vi "Load Config Data MHL CODE.vi"(8 "error in (no error)":errorcluster, 11 "Settings in":refnum<class "Settings.lvclass">) -> (0 "error out":errorcluster, 2 "Config Data":T1={"DS First Launch"=FALSE, "LogBaseFolder"=path "", "Live Logging"=FALSE, "Server Port"=0, "Max Number ML Rows"=0, "AM.WinBounds"={"Left"=0, "Top"=0, "Right"=0, "Bottom"=0}, "AM.FP.State"=enum."Invalid", "AM.Monitor"=0, "AM.Column Widths"=[], "ML.Visible Columns"=[], "ML.Splitter Position"=0, "ML.Column Widths"=[], "ML.WinBounds"={"Left"=0, "Top"=0, "Right"=0, "Bottom"=0}, "ML.FP.State"=enum."Invalid", "ML.Monitor"=0}, 3 "Settings out":refnum<class "Settings.lvclass">)   [LabVIEW 2017, in "Settings.lvclass"]
uses:
  Settings.lvclass
  Config Data.ctl
  <vilib>/Utility/miscctls.llb/LVRectTypeDef.ctl
  <vilib>/Utility/miscctls.llb/LVAllMonitorsDisplayTypeDef.ctl
  <vilib>/Utility/config.llb/Read Key (Boolean).vi
  <vilib>/Utility/config.llb/Read Key (Path).vi
  <vilib>/Utility/config.llb/Read Key (U32).vi
  <vilib>/Utility/config.llb/Read Key (String).vi
  <vilib>/Utility/config.llb/Read Key (I32).vi
  <vilib>/Utility/config.llb/NI_LVConfig.lvlib
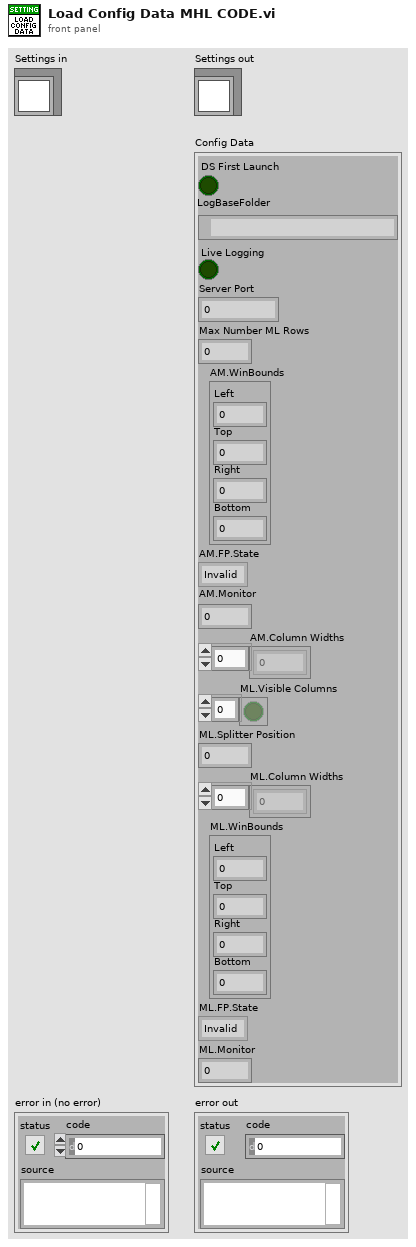
[diagram p1: front panel]
types:
  T1 = typedef "Settings.lvclass/Config Data.ctl" = cluster{"DS First Launch":bool, "LogBaseFolder":path, "Live Logging":bool, "Server Port":u16, "Max Number ML Rows":i32, "AM.WinBounds":T2, "AM.FP.State":enum32{"Invalid", "Standard", "Closed", "Hidden", "Minimized", "Maximized"}, "AM.Monitor":u16, "AM.Column Widths":u32[], "ML.Visible Columns":bool[], "ML.Splitter Position":i32, "ML.Column Widths":u32[], "ML.WinBounds":T2, "ML.FP.State":enum32{"Invalid", "Standard", "Closed", "Hidden", "Minimized", "Maximized"}, "ML.Monitor":u16}
  T2 = typedef "LVRectTypeDef.ctl" = cluster{"Left":i16, "Top":i16, "Right":i16, "Bottom":i16}
  T3 = enum32{"Invalid", "Standard", "Closed", "Hidden", "Minimized", "Maximized"}
  T4 = typedef "LVAllMonitorsDisplayTypeDef.ctl" = cluster{"Bounds":cluster{"Left":i16, "Top":i16, "Right":i16, "Bottom":i16}, "Depth":i16}[]
  T5 = typedef "NI_LVConfig.lvlib/Config Data RefNum.ctl" = refnum<k1>
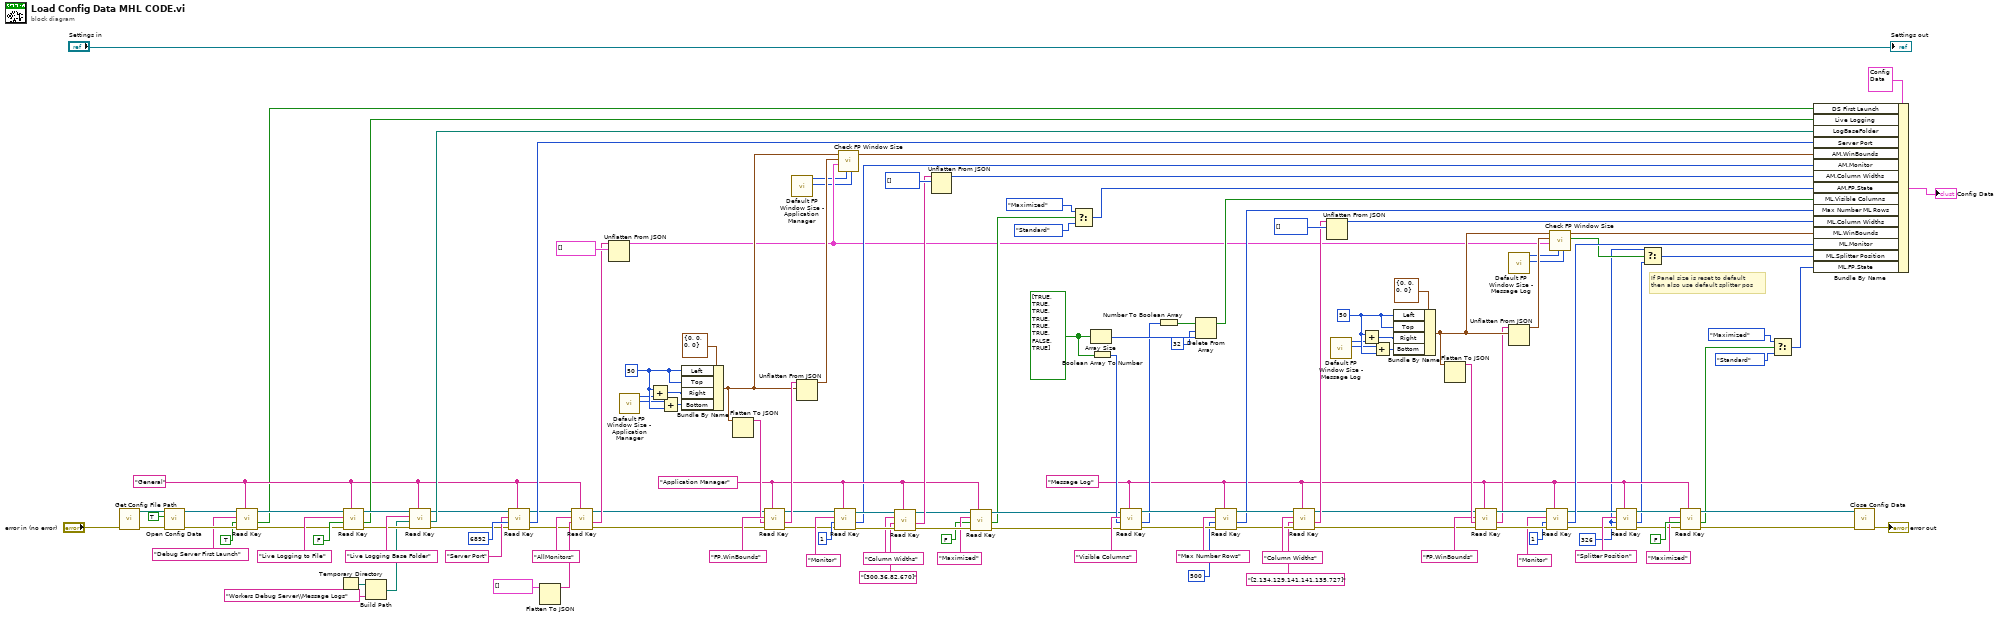
[diagram p0: block diagram]
diagram:
  w11 = 326 ("Splitter Position")
  w39 = i16 50 ("Height")
  w91 = bool[] [TRUE, TRUE, TRUE, TRUE, TRUE, TRUE, FALSE, TRUE] ("Removed ML Columns")
  w105 = i16 50 ("Height")
  w13 = "Message Log" ("section")
  w67 = "Application Manager" ("section")
  w4 = "General" ("section")
  # "If Panel size is reset to default\nthen also use default splitter pos"
  n1 = call "Get Config File Path.vi"("error in (no error)"="error in (no error)") -> ("error out"=w128:errorcluster, "appended path"=w129:path)  [unwired: 9 in]
  n2 = call <vilib>:"Open Config Data.vi"("error in (no error)"=w128, "create file if necessary (T)"=TRUE, "configuration file path"=w129) -> ("error out"=w7:errorcluster, "refnum"=w8:T5)  [unwired: 6 in, 1 out]
  n3 = call-poly <vilib>:"Read Key.vi"("section"=w4, "error in (no error)"=w7, "default value"=TRUE, "key"="Debug Server First Launch" ("name or relative path"), "refnum"=w8) -> ("error out"=w5:errorcluster, "value"=w1:bool, "refnum out"=w6:T5)  [unwired: 3 in, 1 out]
  n4 = Temporary Directory() -> (w119:path)
  n5 = call-poly <vilib>:"Read Key.vi"("section"=w4, "error in (no error)"=w5, "default value"=FALSE, "key"="Live Logging to File", "refnum"=w6) -> ("error out"=w125:errorcluster, "value"=w112:bool, "refnum out"=w126:T5)  [unwired: 3 in, 1 out]
  n6 = Build Path(base path=w119, name or relative path="Workers Debug Server\\Message Logs") -> (appended path=w118:path)
  n7 = call-poly <vilib>:"Read Key.vi"("section"=w4, "error in (no error)"=w125, "default value"=w118, "key"="Live Logging Base Folder", "refnum"=w126) -> ("error out"=w107:errorcluster, "value"=w111:path, "refnum out"=w108:T5)  [unwired: 3 in, 1 out]
  n8 = call-poly <vilib>:"Read Key.vi"("section"=w4, "error in (no error)"=w107, "default value"=u32 6892, "key"="Server Port", "refnum"=w108) -> ("error out"=w55:errorcluster, "value"=w106:u32, "refnum out"=w56:T5)  [unwired: 3 in, 1 out]
  n9 = Flatten To JSON(anything=T4 [] ("Display:All Monitors")) -> (JSON string=w115:string)  [unwired: 2 in, 1 out]
  n10 = call-poly <vilib>:"Read Key.vi"("section"=w4, "error in (no error)"=w55, "default value"=w115, "key"="AllMonitors", "refnum"=w56) -> ("error out"=w54:errorcluster, "value"=w96:string, "refnum out"=w53:T5)  [unwired: 3 in, 1 out]
  n11 = Unflatten From JSON(JSON string=w96, type and defaults=T4 [] ("Display:All Monitors")) -> (value=w25:T4)  [unwired: 5 in, 1 out]
  n12 = call "Default FP Window Size - Application Manager.vi"() -> ("Height"=w101:i16, "Width"=w103:i16)  [unwired: 10 in]
  n13 = Add(x=w105, y=w103) -> (x+y=w104:i16)
  n14 = Add(x=w101, y=w105) -> (x+y=w102:i16)
  n15 = Bundle By Name(cluster=T2 {"Left"=0, "Top"=0, "Right"=0, "Bottom"=0} ("output cluster"), "Left"=w105, "Top"=w105, "Right"=w104, "Bottom"=w102) -> (w68:T2)
  n16 = Flatten To JSON(anything=w68) -> (JSON string=w99:string)  [unwired: 2 in, 1 out]
  n17 = call-poly <vilib>:"Read Key.vi"("section"=w67, "error in (no error)"=w54, "default value"=w99, "key"="FP.WinBounds", "refnum"=w53) -> ("error out"=w52:errorcluster, "value"=w97:string, "refnum out"=w51:T5)  [unwired: 3 in, 1 out]
  n18 = call "Default FP Window Size - Application Manager.vi"() -> ("Height"=w23:i16, "Width"=w24:i16)  [unwired: 10 in]
  n19 = Unflatten From JSON(JSON string=w97, type and defaults=w68) -> (value=w69:T2)  [unwired: 5 in, 1 out]
  n20 = call-poly <vilib>:"Read Key.vi"("section"=w67, "error in (no error)"=w52, "default value"=1 ("Splitter Position"), "key"="Monitor", "refnum"=w51) -> ("error out"=w88:errorcluster, "value"=w65:i32, "refnum out"=w87:T5)  [unwired: 3 in, 1 out]
  n21 = call "Check FP Window Size.vi"("Default Height"=w23, "Default Width"=w24, "All Monitors Display"=w25, "FP.WinBounds"=w69, "Default"=w68) -> ("FP.WinBounds out"=w66:T2)  [unwired: 5 in, 1 out]
  n22 = call-poly <vilib>:"Read Key.vi"("section"=w67, "error in (no error)"=w88, "default value"="[300,36,82,670]", "key"="Column Widths", "refnum"=w87) -> ("error out"=w78:errorcluster, "value"=w81:string, "refnum out"=w76:T5)  [unwired: 3 in, 1 out]
  n23 = Unflatten From JSON(JSON string=w81, type and defaults=u32[] [] ("Column Widths")) -> (value=w64:u32[])  [unwired: 5 in, 1 out]
  n24 = call-poly <vilib>:"Read Key.vi"("section"=w67, "error in (no error)"=w78, "default value"=FALSE, "key"="Maximized", "refnum"=w76) -> ("error out"=w77:errorcluster, "value"=w72:bool, "refnum out"=w75:T5)  [unwired: 3 in, 1 out]
  n25 = Select(t=T3."Maximized" ("y"), s=w72, f=T3."Standard" ("y")) -> (s? t:f=w63:T3)
  n26 = Array Size(array=w91) -> (size(s)=w94:i32)
  n27 = Boolean Array To Number(Boolean array=w91) -> (number=w90:u32)
  n28 = call-poly <vilib>:"Read Key.vi"("section"=w13, "error in (no error)"=w77, "default value"=w90, "key"="Visible Columns", "refnum"=w75) -> ("error out"=w123:errorcluster, "value"=w89:u32, "refnum out"=w124:T5)  [unwired: 3 in, 1 out]
  n29 = Number To Boolean Array(number=w89) -> (Boolean array=w93:bool[])
  n30 = Delete From Array(array=w93, length=32, index=w94) -> (array with subset deleted=w62:bool[])  [unwired: 1 out]
  n31 = call-poly <vilib>:"Read Key.vi"("section"=w13, "error in (no error)"=w123, "default value"=500, "key"="Max Number Rows", "refnum"=w124) -> ("error out"=w83:errorcluster, "value"=w61:i32, "refnum out"=w84:T5)  [unwired: 3 in, 1 out]
  n32 = call-poly <vilib>:"Read Key.vi"("section"=w13, "error in (no error)"=w83, "default value"="[2,134,129,141,141,135,727]", "key"="Column Widths", "refnum"=w84) -> ("error out"=w34:errorcluster, "value"=w79:string, "refnum out"=w33:T5)  [unwired: 3 in, 1 out]
  n33 = Unflatten From JSON(JSON string=w79, type and defaults=u32[] [] ("Column Widths")) -> (value=w60:u32[])  [unwired: 5 in, 1 out]
  n34 = call "Default FP Window Size - Message Log.vi"() -> ("Height"=w21:i16, "Width"=w22:i16)  [unwired: 10 in]
  n35 = Add(x=w39, y=w22) -> (x+y=w40:i16)
  n36 = Add(x=w21, y=w39) -> (x+y=w41:i16)
  n37 = Bundle By Name(cluster=T2 {"Left"=0, "Top"=0, "Right"=0, "Bottom"=0} ("output cluster"), "Left"=w39, "Top"=w39, "Right"=w40, "Bottom"=w41) -> (w48:T2)
  n38 = Flatten To JSON(anything=w48) -> (JSON string=w43:string)  [unwired: 2 in, 1 out]
  n39 = call-poly <vilib>:"Read Key.vi"("section"=w13, "error in (no error)"=w34, "default value"=w43, "key"="FP.WinBounds", "refnum"=w33) -> ("error out"=w49:errorcluster, "value"=w44:string, "refnum out"=w50:T5)  [unwired: 3 in, 1 out]
  n40 = call "Default FP Window Size - Message Log.vi"() -> ("Height"=w19:i16, "Width"=w20:i16)  [unwired: 10 in]
  n41 = Unflatten From JSON(JSON string=w44, type and defaults=w48) -> (value=w47:T2)  [unwired: 5 in, 1 out]
  n42 = call-poly <vilib>:"Read Key.vi"("section"=w13, "error in (no error)"=w49, "default value"=1 ("Splitter Position"), "key"="Monitor", "refnum"=w50) -> ("error out"=w16:errorcluster, "value"=w32:i32, "refnum out"=w17:T5)  [unwired: 3 in, 1 out]
  n43 = call "Check FP Window Size.vi"("Default Height"=w19, "Default Width"=w20, "All Monitors Display"=w25, "FP.WinBounds"=w47, "Default"=w48) -> ("Use Default Values"=w12:bool, "FP.WinBounds out"=w35:T2)  [unwired: 5 in]
  n44 = call-poly <vilib>:"Read Key.vi"("section"=w13, "error in (no error)"=w16, "default value"=w11, "key"="Splitter Position", "refnum"=w17) -> ("error out"=w15:errorcluster, "value"=w10:i32, "refnum out"=w14:T5)  [unwired: 3 in, 1 out]
  n45 = Select(t=w11, s=w12, f=w10) -> (s? t:f=w9:i32)
  n46 = call-poly <vilib>:"Read Key.vi"("section"=w13, "error in (no error)"=w15, "default value"=FALSE, "key"="Maximized", "refnum"=w14) -> ("error out"=w28:errorcluster, "value"=w27:bool, "refnum out"=w29:T5)  [unwired: 3 in, 1 out]
  n47 = Select(t=T3."Maximized" ("y"), s=w27, f=T3."Standard" ("y")) -> (s? t:f=w26:T3)
  n48 = Bundle By Name(cluster=T1 {"DS First Launch"=FALSE, "LogBaseFolder"=path "", "Live Logging"=FALSE, "Server Port"=0, "Max Number ML Rows"=0, "AM.WinBounds"={"Left"=0, "Top"=0, "Right"=0, "Bottom"=0}, "AM.FP.State"=enum."Invalid", "AM.Monitor"=0, "AM.Column Widths"=[], "ML.Visible Columns"=[], "ML.Splitter Position"=0, "ML.Column Widths"=[], "ML.WinBounds"={"Left"=0, "Top"=0, "Right"=0, "Bottom"=0}, "ML.FP.State"=enum."Invalid", "ML.Monitor"=0} ("Data"), "DS First Launch"=w1, "Live Logging"=w112, "LogBaseFolder"=w111, "Server Port"=w106, "AM.WinBounds"=w66, "AM.Monitor"=w65, "AM.Column Widths"=w64, "AM.FP.State"=w63, "ML.Visible Columns"=w62, "Max Number ML Rows"=w61, "ML.Column Widths"=w60, "ML.WinBounds"=w35, "ML.Monitor"=w32, "ML.Splitter Position"=w9, "ML.FP.State"=w26) -> (→"Config Data":T1)
  n49 = call <vilib>:"Close Config Data.vi"("error in (no error)"=w28, "refnum"=w29) -> ("error out"=→"error out":errorcluster)  [unwired: 8 in, 1 out]
  "Settings out" <- "Settings in"
